vi "MetodoGET.vi"(0 "Sinal":string, 1 "LabVIEW Web Service Request":refnum<class "Web Request.lvclass">, 5 "Tempo":dbl min=0.0, 7 "Offset":dbl min=-10.0 max=10.0, 9 "Amplitude":dbl min=0.0 max=10.0, 11 "Fase":dbl) -> ()   [LabVIEW 2020]
uses:
  <vilib>/wsapi/Web Request.lvclass
  5bb1ef98-1994-4d65-9c78-bc6588d51ed2.vi
panel:
  # "Use the Web Service Request input terminal to call the VIs on the Web Services palette. Do not remove it from the connector pane unless you don't need access to the palette."
  # "Each additional control wired to the connector pane will be available as an input in the URL. To include an indicator in terminal-mode output (the default setting), it must also be wired to the connector pane."
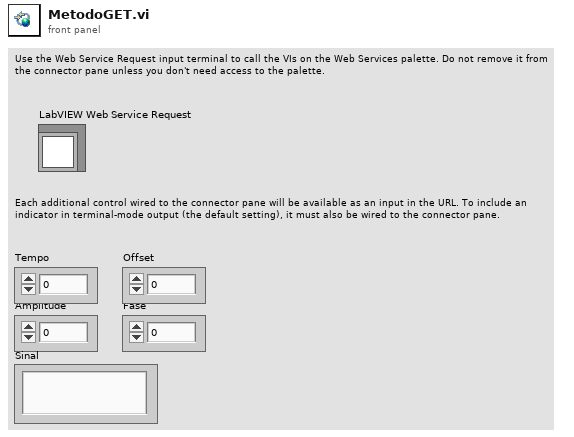
[diagram p1: front panel]
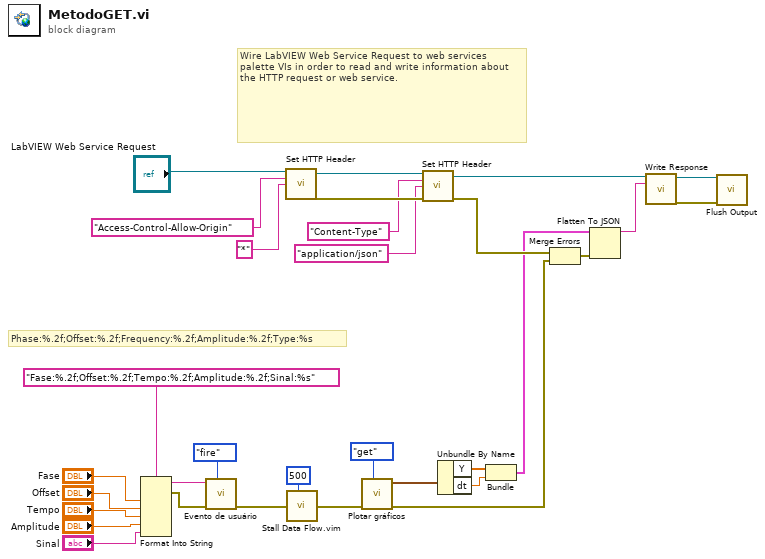
[diagram p0: block diagram]
diagram:
  # "Phase:%.2f;Offset:%.2f;Frequency:%.2f;Amplitude:%.2f;Type:%s"
  # "Wire LabVIEW Web Service Request to web services palette VIs in order to read and write information about the HTTP request or web service."
  n1 = Format Into String(format string="Fase:%.2f;Offset:%.2f;Tempo:%.2f;Amplitude:%.2f;Sinal:%s", "Fase", "Offset", "Tempo", "Amplitude", "Sinal") -> (resulting string=w13:string, error out=w9:errorcluster)  [unwired: 2 in]
  n2 = call "Evento de usuário.vi"("Enum"=enum16{"create", "fire", "destroy"}."fire", "error in (no error)"=w9, "Dados da onda"=w13) -> ("error out"=w12:errorcluster)  [unwired: 7 in, 1 out]
  n3 = call <vilib>:"Set HTTP Header.vi"("LabVIEW Web Service Request"="LabVIEW Web Service Request", "header"="Access-Control-Allow-Origin", "header value"="*") -> ("LabVIEW Web Service Request out"=w31:refnum<class "Web Request.lvclass">, "error out"=w30:errorcluster)  [unwired: 11 in]
  n4 = call "Stall Data Flow.vim"("value in"=w12, "milliseconds to wait"=u32 500) -> ("value out"=w11:errorcluster)  [unwired: 1 out]
  n5 = call "Plotar gráficos.vi"("Enum"=enum16{"set", "get"}."get", "error in (no error)"=w11) -> ("error out"=w6:errorcluster, "Plot"=w2:waveform(dbl))  [unwired: 8 in]
  n6 = call <vilib>:"Set HTTP Header.vi"("LabVIEW Web Service Request"=w31, "header"="Content-Type", "header value"="application/json", "error in (no error)"=w30) -> ("LabVIEW Web Service Request out"=w29:refnum<class "Web Request.lvclass">, "error out"=w5:errorcluster)  [unwired: 10 in]
  n7 = Unbundle By Name(w2) -> ("Y"=w4:dbl[], "dt"=w3:dbl)
  n8 = Bundle("Y"=w4, "dt"=w3) -> (w1:cluster{"Y":dbl[], "dt":dbl})  [unwired: 1 in]
  n9 = Merge Errors(w5, w6) -> (w7:errorcluster)
  n10 = Flatten To JSON(anything=w1, error in (no error)=w7) -> (JSON string=w21:string)  [unwired: 1 in, 1 out]
  n11 = call <vilib>:"Write Response.vi"("LabVIEW Web Service Request"=w29, "response string"=w21) -> ("LabVIEW Web Service Request out"=w23:refnum<class "Web Request.lvclass">, "error out"=w22:errorcluster)  [unwired: 12 in]
  n12 = call <vilib>:"Flush Output.vi"("LabVIEW Web Service Request"=w23, "error in (no error)"=w22) -> ()  [unwired: 12 in, 2 out]
